vi "UI Main.vi"() -> ()   [LabVIEW 2018]
uses:
  robot state.ctl
  internalstate.ctl
  TrialListElements.ctl
  trial type.ctl
  rewtype.ctl
  frontpanelrobotparams.ctl
  commands.ctl
  DataRecord.ctl
  TrialParams.ctl
  <vilib>/Utility/file.llb/Write Delimited Spreadsheet (DBL).vi
  <resource>/objmgr/ni.dex.rc
panel:
  out "Ready to exit":bool
  in  "nocurrent":bool
  in  "Exit":bool
  in  "Robot\nparameters":T1
  in  "CurrentParams":T2={"TrialType"=enum."2D aiming", "Angle"=0.0, "Length"=0.0, "TurnLength"=0.0, "TurnAngle"=0.0, "MaxError"=0.0, "RewardScale"=0.0, "Timeout"=100, "RewardType"=enum."Normal"} caption="Current trial parameters"
  out "Completed":bool caption="Last trial\ncompleted"
  out "Advance trial":bool
  out "Current reward":u32
  in  "waitforcompletion":bool caption="Wait for \ncompletion"
  out "Last trial rewarded":bool
  in  "AdvanceOnReward":bool=TRUE caption="Only advance\nafter reward"
  in  "Rewarded length":sgl=6.0
  in  "Trial List":T2[](array[typedef]) caption="Upcoming trials"
  in  "Reward":i32=70 caption="Reward (ms)"
  in  "Give reward":bool
  out "Targpos":sgl[](array[numeric])
  in  "Trial list file":path=path "C:/Users/cnc/Desktop/Robot_visual_050319/trial lists/clamp0.csv"
  in  "data file":path=path "C:/Users/cnc/Desktop/junk.csv" caption="Data record file"
  in  "Write data":bool
  out "Last\nmovement":dbl=0.1 caption="Last trial\nradial length" format="%#_2g"
  out "Last lateral\ndeviation":dbl=0.1 caption="Last trial\nlateral length" format="%#.2g"
  out "rewards":i32 caption="# of Rewards"
  in  "Stop block":bool
  out "Xpos":sgl format="%#_3g"
  out "Ypos":sgl=56.0 format="%#_3g"
  in  "Start block":bool
  out "loaded":bool caption="Loaded a\ntrial list"
  out "movement number":i32 caption="Trial #"
  out "Last event":i32 format="%.0e"
  out "UI state":T5
  out "Trial started":bool
  in  "Go to target":bool
  in  "X home":sgl
  in  "Y home":sgl=56.0
  out "Robot state":T6=enum."Go somewhere"
  in  "Hold position":bool
  out "Homing":bool
  in  "Find home":bool
  in  "Go home":bool
  in  "X target":sgl
  in  "Y target":sgl=56.0
  in  "Enable drives":bool
  # "Movement criteria"
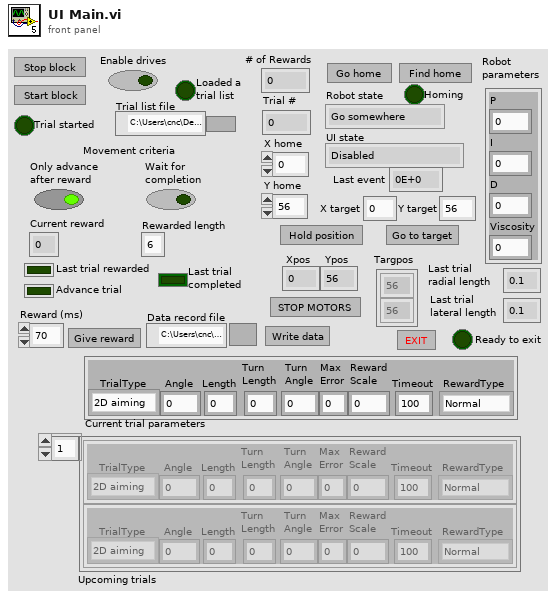
[diagram p1: front panel]
types:
  T1 = typedef "frontpanelrobotparams.ctl" = cluster{"Kp":dbl, "Bp":dbl, "Ip":dbl, "Viscosity":dbl}
  T2 = typedef "TrialListElements.ctl" = cluster{"TrialType":T3, "Angle":dbl, "Length":dbl, "TurnLength":dbl, "TurnAngle":dbl, "MaxError":dbl, "RewardScale":dbl, "Timeout":i32, "RewardType":T4}
  T3 = typedef "trial type.ctl" = enum8{"Linear", "2D aiming", "Two-part"}
  T4 = typedef "rewtype.ctl" = enum16{"Normal", "No reward"}
  T5 = typedef "internalstate.ctl" = enum16{"Disabled", "Waiting for movement", "Moving", "Post-trial", "Returning handle", "Starting trial", "Post-reward"}
  T6 = typedef "robot state.ctl" = enum16{"Hold", "Movement", "Homing", "Go somewhere", "Go home", "Disabled"}
  T7 = typedef "DataRecord.ctl" = cluster{"X":sgl, "Y":sgl, "MotorCurrent1":i16, "MotorCurrent2":i16, "TrialType":T3, "Angle":sgl, "FrameCnt1":i16, "FrameCnt2":i16, "Licking":bool, "Solenoid":bool, "robot state":T6}
  T8 = typedef "commands.ctl" = enum16{"TrialParams", "X home", "Y home", "Target X", "Target Y", "Enable drives", "Robot state", "Shut down", "Reward duration", "Start reward"}
  T9 = typedef "TrialParams.ctl" = cluster{"Kp":dbl, "Bp":dbl, "Ip":dbl, "TrialType":T3, "Angle":dbl, "Viscosity":dbl, "Length":dbl, "MaxError":dbl, "TurnLength":dbl, "TurnAngle":dbl}
  T10 = cluster{"Kp":dbl, "Bp":dbl, "Ip":dbl, "Viscosity":dbl}
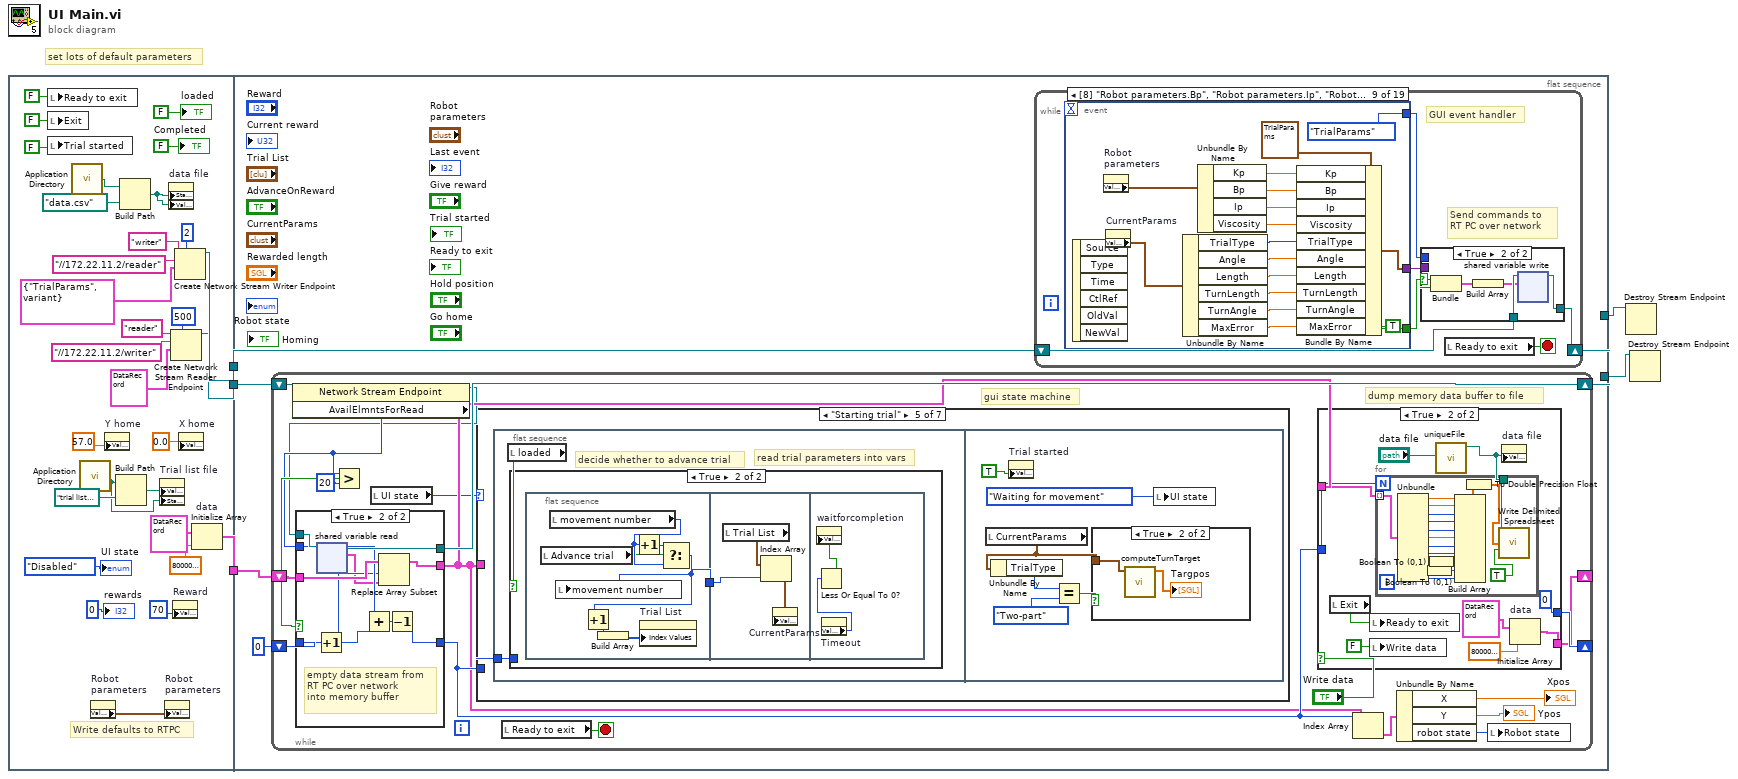
[diagram p0: block diagram]
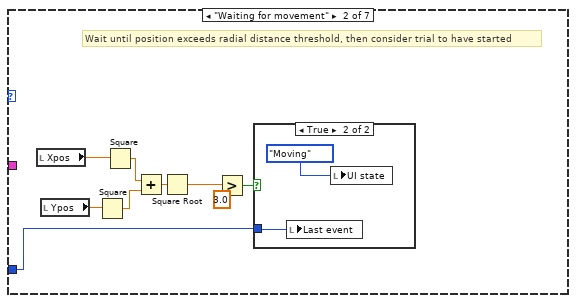
[diagram p3: hidden frame]
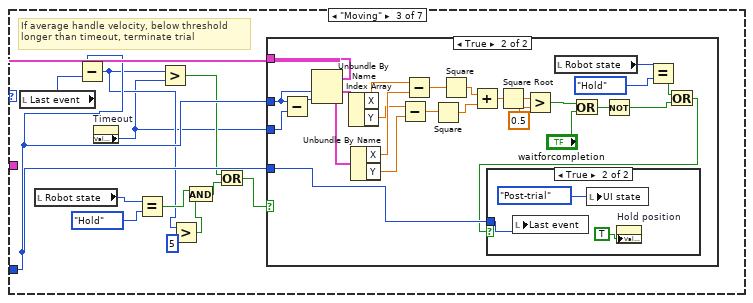
[diagram p5: hidden frame]
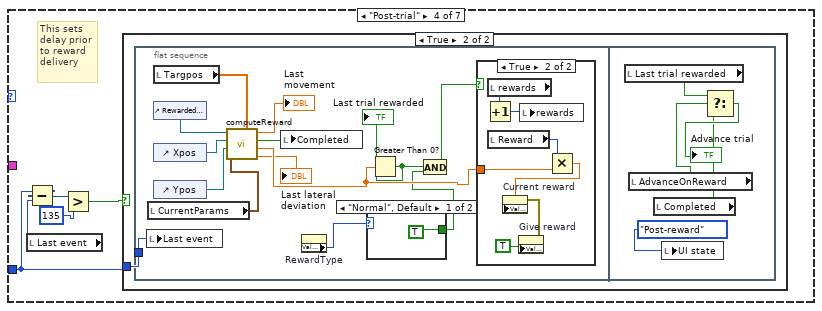
[diagram p8: hidden frame]
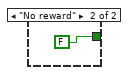
[diagram p10: hidden frame]
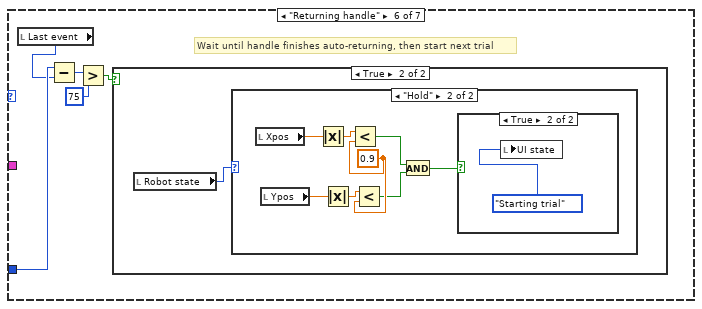
[diagram p14: hidden frame]
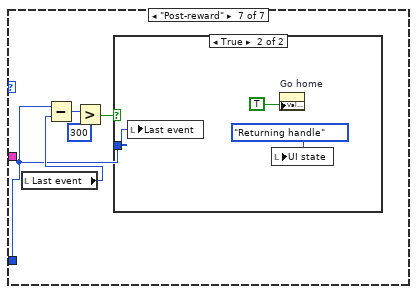
[diagram p18: hidden frame]
diagram:
  # "set lots of default parameters"
  n1 = flat-sequence {
    tunnel: [w28] -> w5
    tunnel: [w27] -> w4
    tunnel: [w25] -> w3
    tunnel: w5 -> [w41]
    tunnel: w4 -> [w40]
    tunnel: [w39] -> w2
    tunnel: w3 -> [w38]
    tunnel: [w36] -> w1
    frame #0 {
      # "Write defaults to RTPC"
      n2 = local write "Ready to exit"(FALSE) -> ()
      n3 = local write "Exit"(FALSE) -> ()
      n4 = local write "Trial started"(FALSE) -> ()
      n5 = call <vilib>:"Application Directory.vi"() -> ("Application Directory"=w19:path)
      n6 = call <vilib>:"Application Directory.vi"() -> ("Application Directory"=w7:path)
      n7 = property on="Robot\nparameters" class="Clust (strict)"() -> ("Value"=w6:T10)  [unwired: 2 in, 2 out]
      n8 = property on="Y home" class="DigNum (strict)"("Val(Sgnl)"=sgl 57.0) -> ()  [unwired: 2 in, 2 out]
      n9 = Build Path(base path=w7, name or relative path=path "trial lists/2D_0deg.csv") -> (appended path=w13:path)
      n10 = Build Path(base path=w19, name or relative path=path "data.csv") -> (appended path=w8:path)
      n11 = property on="Trial list file" class="Path"("Val(Sgnl)"=w13, "StartPath"=w7) -> ()  [unwired: 2 in, 2 out]
      n12 = property on="Robot\nparameters" class="Clust (strict)"("Val(Sgnl)"=w6) -> ()  [unwired: 2 in, 2 out]
      n13 = property on="data file" class="Path"("StartPath"=w8, "Val(Sgnl)"=w8) -> ()  [unwired: 2 in, 2 out]
      n14 = Create Network Stream Reader Endpoint(7:500, 9:T7 {"X"=0.0, "Y"=0.0, "MotorCurrent1"=0, "MotorCurrent2"=0, "TrialType"=enum."Linear", "Angle"=0.0, "FrameCnt1"=0, "FrameCnt2"=0, "Licking"=FALSE, "Solenoid"=FALSE, "robot state"=enum."Go somewhere"} ("DataRecord"), 10:"//172.22.11.2/writer", 11:"reader") -> (3:w27:refnum<k21>)  [unwired: 3 in, 1 out]
      n15 = property on="Reward" class="DigNum (strict)"("Val(Sgnl)"=70) -> ()  [unwired: 2 in, 2 out]
      n16 = Create Network Stream Writer Endpoint(7:2, 9:cluster{"Commands":T8, variant} {"Commands"=enum."TrialParams", variant}, 10:"//172.22.11.2/reader", 11:"writer") -> (3:w28:refnum<k21>)  [unwired: 3 in, 1 out]
      n17 = property on="X home" class="DigNum (strict)"("Val(Sgnl)"=sgl 0.0) -> ()  [unwired: 2 in, 2 out]
      n18 = Initialize Array "data"(T7 {"X"=0.0, "Y"=0.0, "MotorCurrent1"=0, "MotorCurrent2"=0, "TrialType"=enum."Linear", "Angle"=0.0, "FrameCnt1"=0, "FrameCnt2"=0, "Licking"=FALSE, "Solenoid"=FALSE, "robot state"=enum."Go somewhere"} ("DataRecord"), sgl 8000000.0) -> (w25:T7[])
      "loaded" <- FALSE
      "rewards" <- 0
      "Completed" <- FALSE
      "UI state" <- internalstate."Disabled" ("internal state")
    }
    frame #1 {
      n19 = while {
        shift-right: [w59] -> w39
        shift-left: w40 -> [w60]
        shift-right: [w55] -> _
        shift-left: 0 -> [w56]
        shift-right: [w43] -> _
        shift-left: w38 -> [w57]
        stop <- w58 stop-if-true
        # "gui state machine"
        # "dump memory data buffer to file"
        n20 = property class="Network Stream Endpoint"(reference=w60) -> (reference out=w49:refnum<k21>, "AvailElmntsForRead"=w52:i32)  [unwired: 1 in, 1 out]
        n21 = Greater?(x=w52, y=20) -> (0:w53:bool)
        n22 = case shown="True" w53 {
          tunnel: w52 -> [_ w232]
          tunnel: w49 -> [w226 w236]
          tunnel: [w226 w235] -> w59
          tunnel: w57 -> [w225 w234]
          tunnel: w56 -> [w224 w231]
          tunnel: [w225 w233] -> w50
          tunnel: [w224 w228] -> w54
          frame False {
          }
          frame True {
            # "empty data stream from\nRT PC over network\ninto memory buffer"
            n23 = Increment(x=w231) -> (x+1=w229:i32)
            n24 = shared-variable-read(w236, w232) -> (w235:refnum<k21>, w227:T7[])  [unwired: 2 in, 2 out]
            n25 = Add(x=w232, y=w229) -> (x+y=w230:i32)
            n26 = Replace Array Subset(array=w234, new element=w227, index=w229) -> (w233:T7[])
            n27 = Decrement(x=w230) -> (x-1=w228:i32)
          }
        }
        n28 = local read "UI state"() -> (w48:T5)
        n29 = case shown="\"Starting trial\"" w48 {
          tunnel: w50 -> [_ _ w83 _ _ _ _]
          tunnel: w54 -> [_ w64 w82 w115 w148 w174 w186]
          frame "Disabled", Default {
          }
          frame "Waiting for movement" {
            # "Wait until position exceeds radial distance threshold, then consider trial to have started"
            n30 = local read "Xpos"() -> (w62:sgl)
            n31 = local read "Ypos"() -> (w61:sgl)
            n32 = Square(x=w61) -> (x^2=w68:sgl)
            n33 = Square(x=w62) -> (x^2=w69:sgl)
            n34 = Add(x=w69, y=w68) -> (x+y=w67:sgl)
            n35 = Square Root(x=w67) -> (sqrt(x)=w66:sgl)
            n36 = Greater?(x=w66, y=sgl 3.0) -> (0:w63:bool)
            n37 = case shown="True" w63 {
              tunnel: w64 -> [_ w70]
              frame False {
              }
              frame True {
                n38 = local write "Last event"(w70) -> ()
                n39 = local write "UI state"(internalstate."Moving" ("internal state")) -> ()
              }
            }
          }
          frame "Moving" {
            # "If average handle velocity, below threshold \nlonger than timeout, terminate trial"
            n40 = local read "Last event"() -> (w84:i32)
            n41 = local read "Robot state"() -> (w80:T6)
            n42 = Subtract(x=w82, y=w84) -> (x-y=w76:i32)
            n43 = property on="Timeout" class="DigNum (strict)"() -> ("Value"=w72:i32)  [unwired: 2 in, 2 out]
            n44 = Equal?(x=w80, y=robot_state."Hold" ("robot state")) -> (x = y?=w78:bool)
            n45 = Greater?(x=w76, y=w72) -> (0:w79:bool)
            n46 = Greater?(x=w76, y=5) -> (0:w77:bool)
            n47 = And(x=w78, y=w77) -> (x .and. y?=w74:bool)
            n48 = Or(x=w79, y=w74) -> (x .or. y?=w73:bool)
            n49 = case shown="True" w73 {
              tunnel: w83 -> [_ w93]
              tunnel: w72 -> [_ w98]
              tunnel: w82 -> [_ w102]
              tunnel: w82 -> [_ w92]
              frame False {
              }
              frame True {
                n50 = Subtract(x=w92, y=w98) -> (x-y=w91:i32)
                n51 = Index Array(array=w93, index #1=w92, index #2=w91) -> (element #1=w90:T7, element #2=w89:T7)
                n52 = Unbundle By Name(w90) -> ("X"=w87:sgl, "Y"=w86:sgl)
                n53 = Unbundle By Name(w89) -> ("X"=w88:sgl, "Y"=w85:sgl)
                n54 = Subtract(x=w86, y=w85) -> (x-y=w105:sgl)
                n55 = Subtract(x=w87, y=w88) -> (x-y=w104:sgl)
                n56 = Square(x=w105) -> (x^2=w107:sgl)
                n57 = Square(x=w104) -> (x^2=w106:sgl)
                n58 = Add(x=w106, y=w107) -> (x+y=w108:sgl)
                n59 = Square Root(x=w108) -> (sqrt(x)=w109:sgl)
                n60 = Greater?(x=w109, y=sgl 0.5) -> (0:w103:bool)
                n61 = local read "Robot state"() -> (w99:T6)
                n62 = Or(x=w103, y="waitforcompletion") -> (x .or. y?=w95:bool)
                n63 = Not(x=w95) -> (.not. x?=w94:bool)
                n64 = Equal?(x=w99, y=robot_state."Hold" ("robot state")) -> (x = y?=w100:bool)
                n65 = Or(x=w100, y=w94) -> (x .or. y?=w97:bool)
                n66 = case shown="True" w97 {
                  tunnel: w102 -> [_ w112]
                  frame False {
                  }
                  frame True {
                    n67 = local write "Last event"(w112) -> ()
                    n68 = local write "UI state"(internalstate."Post-trial" ("internal state")) -> ()
                    n69 = property on="Hold position" class="Bool (strict)"("Val(Sgnl)"=TRUE) -> ()  [unwired: 2 in, 2 out]
                  }
                }
              }
            }
          }
          frame "Post-trial" {
            # "This sets\ndelay prior\nto reward\ndelivery"
            n70 = local read "Last event"() -> (w118:i32)
            n71 = Subtract(x=w115, y=w118) -> (x-y=w117:i32)
            n72 = Greater?(x=w117, y=135) -> (0:w116:bool)
            n73 = case shown="True" w116 {
              tunnel: w115 -> [_ w119]
              frame False {
              }
              frame True {
                n74 = flat-sequence {
                  tunnel: w119 -> [w130]
                  frame #0 {
                    n75 = local write "Last event"(w130) -> ()
                    n76 = local read "CurrentParams"() -> (w121:T2)
                    n77 = local read "Targpos"() -> (w123:sgl[])
                    n78 = control-ref of="Rewarded length"() -> (w128:refnum<vi>)
                    n79 = control-ref of="Xpos"() -> (w129:refnum<vi>)
                    n80 = control-ref of="Ypos"() -> (w122:refnum<vi>)
                    n81 = call "computeReward.vi"("RewardedLength"=w128, "X"=w129, "Y"=w122, "TrialListElements"=w121, "targpos"=w123) -> ("ylen"=→"Last\nmovement":dbl, "completed"=w126:bool, "reward"=w133:dbl, "xlen"=→"Last lateral\ndeviation":dbl)  [unwired: 2 in]
                    n82 = local write "Completed"(w126) -> ()
                    n83 = property on="RewardType" class="Enum (strict)"() -> ("Value"=w120:T4)  [unwired: 2 in, 2 out]
                    n84 = case shown="\"Normal\", Default" w120 {
                      tunnel: [TRUE FALSE] -> w125
                      frame "Normal", Default {
                      }
                      frame "No reward" {
                      }
                    }
                    n85 = Greater Than 0?(x=w133) -> (x > 0?=w131:bool)
                    "Last trial rewarded" <- w131
                    n86 = And(x=w131, y=w125) -> (x .and. y?=w132:bool)
                    n87 = case shown="True" w132 {
                      tunnel: w133 -> [_ w138]
                      frame False {
                      }
                      frame True {
                        n88 = local read "rewards"() -> (w141:i32)
                        n89 = Increment(x=w141) -> (x+1=w142:i32)
                        n90 = local read "Reward"() -> (w137:i32)
                        n91 = local write "rewards"(w142) -> ()
                        n92 = Multiply(x=w137, y=w138) -> (x*y=w136:dbl)
                        n93 = property on="Current reward" class="DigNum (strict)"("Val(Sgnl)"=w136) -> (error out=w139:errorcluster)  [unwired: 2 in, 1 out]
                        n94 = property on="Give reward" class="Bool (strict)"(error in=w139, "Val(Sgnl)"=TRUE) -> ()  [unwired: 1 in, 2 out]
                      }
                    }
                  }
                  frame #1 {
                    n95 = local read "Last trial rewarded"() -> (w143:bool)
                    n96 = local read "AdvanceOnReward"() -> (w145:bool)
                    n97 = local read "Completed"() -> (w144:bool)
                    n98 = local write "UI state"(internalstate."Post-reward" ("internal state")) -> ()
                    n99 = Select(t=w143, s=w145, f=w144) -> (s? t:f=→"Advance trial":bool)
                  }
                }
              }
            }
          }
          frame "Starting trial" {
            n100 = flat-sequence {
              tunnel: w148 -> [w149]
              frame #0 {
                # "decide whether to advance trial"
                # "read trial parameters into vars"
                n101 = local read "loaded"() -> (w150:bool)
                n102 = case shown="True" w150 {
                  tunnel: w149 -> [_ _]
                  frame False {
                  }
                  frame True {
                    n103 = flat-sequence {
                      tunnel: [w153] -> w151
                      tunnel: w151 -> [w159]
                      frame #0 {
                        n104 = local read "Advance trial"() -> (w152:bool)
                        n105 = local read "movement number"() -> (w156:i32)
                        n106 = Increment(x=w156) -> (x+1=w157:i32)
                        n107 = Select(t=w157, s=w152, f=w156) -> (s? t:f=w153:i32)
                        n108 = local write "movement number"(w153) -> ()
                        n109 = Increment(x=w153) -> (x+1=w154:i32)
                        n110 = Build Array(w154) -> (w155:i32[])
                        n111 = property on="Trial List" class="Arr (strict)"("Index Values"=w155) -> ()  [unwired: 2 in, 2 out]
                      }
                      frame #1 {
                        n112 = local read "Trial List"() -> (w158:T2[])
                        n113 = Index Array(array=w158, index=w159) -> (element=w160:T2)
                        n114 = property on="CurrentParams" class="Clust (strict)"("Val(Sgnl)"=w160) -> ()  [unwired: 2 in, 2 out]
                      }
                      frame #2 {
                        n115 = property on="Timeout" class="DigNum (strict)"() -> ("Value"=w161:i32)  [unwired: 2 in, 2 out]
                        n116 = Less Or Equal To 0?(x=w161) -> (x <= 0?=w162:bool)
                        n117 = property on="waitforcompletion" class="Bool (strict)"("Val(Sgnl)"=w162) -> ()  [unwired: 2 in, 2 out]
                      }
                    }
                  }
                }
              }
              frame #1 {
                n118 = local read "CurrentParams"() -> (w163:T2)
                n119 = Unbundle By Name(w163) -> ("TrialType"=w164:T3)
                n120 = property on="Trial started" class="Bool (strict)"("Val(Sgnl)"=TRUE) -> ()  [unwired: 2 in, 2 out]
                n121 = Equal?(x=w164, y=trial_type."Two-part" ("Enum")) -> (x = y?=w167:bool)
                n122 = case shown="True" w167 {
                  tunnel: w163 -> [_ w169]
                  frame False {
                  }
                  frame True {
                    n123 = call "computeTurnTarget.vi"("Cluster in"=w169) -> ("Targpos"=→"Targpos":sgl[])  [unwired: 10 in]
                  }
                }
                n124 = local write "UI state"(internalstate."Waiting for movement" ("internal state")) -> ()
              }
            }
          }
          frame "Returning handle" {
            # "Wait until handle finishes auto-returning, then start next trial"
            n125 = local read "Last event"() -> (w173:i32)
            n126 = Subtract(x=w174, y=w173) -> (x-y=w172:i32)
            n127 = Greater?(x=w172, y=75) -> (0:w171:bool)
            n128 = case shown="True" w171 {
              frame False {
              }
              frame True {
                n129 = local read "Robot state"() -> (w176:T6)
                n130 = case shown="\"Hold\"" w176 {
                  frame "Go home", Default {
                  }
                  frame "Hold" {
                    w180 = 0.9
                    n131 = local read "Xpos"() -> (w184:sgl)
                    n132 = local read "Ypos"() -> (w183:sgl)
                    n133 = Absolute Value(x=w184) -> (abs(x)=w182:sgl)
                    n134 = Absolute Value(x=w183) -> (abs(x)=w181:sgl)
                    n135 = Less?(x=w182, y=w180) -> (x < y?=w179:bool)
                    n136 = Less?(x=w181, y=w180) -> (x < y?=w178:bool)
                    n137 = And(x=w179, y=w178) -> (x .and. y?=w177:bool)
                    n138 = case shown="True" w177 {
                      frame False {
                      }
                      frame True {
                        n139 = local write "UI state"(internalstate."Starting trial" ("internal state")) -> ()
                      }
                    }
                  }
                }
              }
            }
          }
          frame "Post-reward" {
            n140 = local read "Last event"() -> (w189:i32)
            n141 = Subtract(x=w186, y=w189) -> (x-y=w188:i32)
            n142 = Greater?(x=w188, y=300) -> (0:w187:bool)
            n143 = case shown="True" w187 {
              tunnel: w186 -> [_ w193]
              frame False {
              }
              frame True {
                n144 = local write "Last event"(w193) -> ()
                n145 = local write "UI state"(internalstate."Returning handle" ("internal state")) -> ()
                n146 = property on="Go home" class="Bool (strict)"("Val(Sgnl)"=TRUE) -> ()  [unwired: 2 in, 2 out]
              }
            }
          }
        }
        n147 = local read "Ready to exit"() -> (w58:bool)
        n148 = case shown="True" "Write data" {
          tunnel: w50 -> [w194 w199]
          tunnel: [w194 w201] -> w43
          tunnel: [w195 0] -> w55
          tunnel: w54 -> [w195 w197]
          frame False {
          }
          frame True {
            n149 = local read "Exit"() -> (w198:bool)
            n150 = local write "Ready to exit"(w198) -> ()
            n151 = local write "Write data"(FALSE) -> ()
            n152 = call "uniqueFile.vi"("PathIn"="data file") -> ("PathOut"=w196:path)  [unwired: 10 in]
            n153 = for {
              N: w197 -> [_]
              tunnel: w199 -> [w223] mode=indexing
              tunnel: w196 -> [w208]
              n154 = Unbundle(w223) -> ("X"=w222:sgl, "Y"=w221:sgl, "MotorCurrent1"=w220:i16, "MotorCurrent2"=w219:i16, "TrialType"=w218:T3, "Angle"=w217:sgl, "FrameCnt1"=w216:i16, "FrameCnt2"=w215:i16, "Licking"=w214:bool, "Solenoid"=w212:bool, "robot state"=w210:T6)
              n155 = Boolean To (0,1)(Boolean=w212) -> (0, 1=w211:i16)
              n156 = Boolean To (0,1)(Boolean=w214) -> (0, 1=w213:i16)
              n157 = Build Array(w222, w221, w220, w219, w218, w217, w216, w215, w213, w211, w210) -> (w209:sgl[])
              n158 = To Double Precision Float(number=w209) -> (double precision float=w207:dbl[])
              n159 = call-poly <vilib>:"Write Delimited Spreadsheet.vi"("file path (dialog if empty)"=w208, "1D data"=w207, "append to file? (new file:F)"=TRUE) -> ()  [unwired: 11 in, 2 out]
            }
            n160 = property on="data file" class="Path"("Val(Sgnl)"=w196) -> ()  [unwired: 2 in, 2 out]
            n161 = Initialize Array "data"(T7 {"X"=0.0, "Y"=0.0, "MotorCurrent1"=0, "MotorCurrent2"=0, "TrialType"=enum."Linear", "Angle"=0.0, "FrameCnt1"=0, "FrameCnt2"=0, "Licking"=FALSE, "Solenoid"=FALSE, "robot state"=enum."Go somewhere"} ("DataRecord"), sgl 8000000.0) -> (w201:T7[])
          }
        }
        n162 = Index Array(array=w50, index=w54) -> (element=w47:T7)
        n163 = Unbundle By Name(w47) -> ("X"=→"Xpos":sgl, "Y"=→"Ypos":sgl, "robot state"=w46:T6)
        n164 = local write "Robot state"(w46) -> ()
      }
      n165 = while {
        shift-right: [w239] -> w36
        shift-left: w41 -> [w242]
        stop <- w238 stop-if-true
        # "GUI event handler"
        # "Send commands to \nRT PC over network"
        n166 = event shown="[8] \"Robot parameters.Bp\", \"Robot parameters.Ip\", \"Robot parameters.Viscosity\", \"CurrentParams.Length\", \"CurrentParams.RewardScale\", \"CurrentParams.TrialType\", \"CurrentParams.Angle\", \"CurrentParams.TurnLength\", \"CurrentParams.TurnAngle\", \"CurrentParams.MaxError\": Value Change" {
          selector: _ -> [_ _ _ _ _ _ _ _ _ _ _ _ _ _ _ _ _ _ _]
          dyn-events: _ -> [_ _ _ _ _ _ _ _ _ _ _ _ _ _ _ _ _ _ _]
          timeout: _ -> [_ _ _ _ _ _ _ _ _ _ _ _ _ _ _ _ _ _ _]
          tunnel: ["Enable drives" robot_state."Go somewhere" ("robot state") robot_state."Movement" ("robot state") "X home" "Y home" TRUE w272 _ w276 w293 _ "X target" "Y target" robot_state."Go home" ("robot state") robot_state."Homing" ("robot state") robot_state."Hold" ("robot state") _ _ _] -> w240
          tunnel: [commands."Enable drives" ("Commands") commands."Robot state" ("Commands") commands."Robot state" ("Commands") commands."X home" ("Commands") commands."Y home" ("Commands") commands."Start reward" ("Commands") commands."Reward duration" ("Commands") _ commands."TrialParams" ("Commands") commands."Robot state" ("Commands") _ commands."Target X" ("Commands") commands."Target Y" ("Commands") commands."Robot state" ("Commands") commands."Robot state" ("Commands") commands."Robot state" ("Commands") _ _ _] -> w241
          tunnel: [TRUE TRUE TRUE TRUE TRUE TRUE TRUE FALSE TRUE TRUE _ TRUE TRUE TRUE TRUE TRUE FALSE FALSE FALSE] -> w237
          event "Enable drives": Value Change {
            n167 = event-data() -> ()  [unwired: 1 in, 5 out]
          }
          event "Go to target": Value Change {
            n168 = event-data() -> ()  [unwired: 1 in, 1 out]
          }
          event "Trial started": Value Change {
            n169 = event-data() -> ()  [unwired: 1 in, 5 out]
            n170 = local write "Trial started"(FALSE) -> ()
          }
          event "X home": Value Change {
            n171 = event-data() -> ()  [unwired: 1 in, 5 out]
          }
          event "Y home": Value Change {
            n172 = event-data() -> ()  [unwired: 1 in, 5 out]
          }
          event "Give reward": Value Change {
            n173 = event-data() -> ()  [unwired: 1 in, 6 out]
            n174 = local write "Give reward"(FALSE) -> ()
          }
          event "Current reward": Value Change {
            n175 = event-data() -> ()  [unwired: 1 in, 6 out]
            n176 = local read "Current reward"() -> (w272:u32)
          }
          event "Reward": Value Change {
            n177 = event-data() -> ()  [unwired: 1 in, 6 out]
            n178 = local read "Reward"() -> (w273:i32)
            n179 = control-ref of="Current reward"() -> (w274:refnum<vi>)
            n180 = property class="DigNum (strict)"(reference=w274, "Val(Sgnl)"=w273) -> ()  [unwired: 1 in, 2 out]
          }
          event Value Change {
            n181 = event-data() -> ()  [unwired: 1 in, 6 out]
            n182 = property on="Robot\nparameters" class="Clust (strict)"() -> ("Value"=w288:T10)  [unwired: 2 in, 2 out]
            n183 = property on="CurrentParams" class="Clust (strict)"() -> ("Value"=w283:T2)  [unwired: 2 in, 2 out]
            n184 = Unbundle By Name(w283) -> ("TrialType"=w282:T3, "Angle"=w281:dbl, "Length"=w280:dbl, "TurnLength"=w279:dbl, "TurnAngle"=w278:dbl, "MaxError"=w277:dbl)
            n185 = Unbundle By Name(w288) -> ("Kp"=w287:dbl, "Bp"=w286:dbl, "Ip"=w285:dbl, "Viscosity"=w284:dbl)
            n186 = Bundle By Name(cluster=T9 {"Kp"=0.0, "Bp"=0.0, "Ip"=0.0, "TrialType"=enum."Linear", "Angle"=0.0, "Viscosity"=0.0, "Length"=0.0, "MaxError"=0.0, "TurnLength"=0.0, "TurnAngle"=0.0} ("TrialParams"), "Kp"=w287, "Bp"=w286, "Ip"=w285, "Viscosity"=w284, "TrialType"=w282, "Angle"=w281, "Length"=w280, "TurnLength"=w279, "TurnAngle"=w278, "MaxError"=w277) -> (w276:T9)
          }
          event "nocurrent": Value Change {
            n187 = event-data() -> ()  [unwired: 1 in, 6 out]
            n188 = local write "UI state"(internalstate."Disabled" ("internal state")) -> ()
            n189 = To Variant(anything=robot_state."Disabled" ("robot state")) -> (Variant=w293:variant)
          }
          event "Exit": Value Change {
            n190 = event-data() -> ()  [unwired: 1 in, 6 out]
            n191 = property on="Write data" class="Bool (strict)"("Val(Sgnl)"="Exit") -> ()  [unwired: 2 in, 2 out]
          }
          event "X target": Value Change {
            n192 = event-data() -> ()  [unwired: 1 in, 5 out]
          }
          event "Y target": Value Change {
            n193 = event-data() -> ()  [unwired: 1 in, 5 out]
          }
          event "Go home": Value Change {
            n194 = event-data() -> ()  [unwired: 1 in, 5 out]
            n195 = local write "Go home"(FALSE) -> ()
          }
          event "Find home": Value Change {
            n196 = event-data() -> ()  [unwired: 1 in, 5 out]
          }
          event "Hold position": Value Change {
            n197 = event-data() -> ()  [unwired: 1 in, 5 out]
            n198 = local write "Hold position"(FALSE) -> ()
          }
          event "Trial list file": Value Change {
            n199 = event-data() -> ()  [unwired: 1 in, 1 out]
            n200 = call "ReadTrialList.vi"("InputList"="Trial list file") -> ("TrialList"=w315:T2[])  [unwired: 10 in]
            n201 = local write "loaded"(TRUE) -> ()
            n202 = property on="Trial List" class="Arr (strict)"("Value"=w315) -> ()  [unwired: 2 in, 2 out]
            "movement number" <- 0
          }
          event "Stop block": Value Change {
            n203 = event-data() -> ()  [unwired: 1 in, 1 out]
            n204 = property on="Hold position" class="Bool (strict)"("Val(Sgnl)"=TRUE) -> ()  [unwired: 2 in, 2 out]
            n205 = local write "UI state"(internalstate."Disabled" ("internal state")) -> ()
          }
          event "Start block": Value Change {
            n206 = event-data() -> ()  [unwired: 1 in, 1 out]
            n207 = local write "UI state"(internalstate."Starting trial" ("internal state")) -> ()
          }
        }
        n208 = case shown="True" w237 {
          tunnel: w242 -> [w243 w249]
          tunnel: w241 -> [_ w248]
          tunnel: w240 -> [_ w247]
          tunnel: [w243 w245] -> w239
          frame False {
          }
          frame True {
            n209 = Bundle("Commands"=w248, "Variant"=w247) -> (w246:cluster{"Commands":T8, "Variant":variant})  [unwired: 1 in]
            n210 = Build Array(w246) -> (w244:cluster{"Commands":T8, "Variant":variant}[])
            n211 = shared-variable-write(w249, w244) -> (w245:refnum<k21>)  [unwired: 2 in, 2 out]
          }
        }
        n212 = local read "Ready to exit"() -> (w238:bool)
      }
    }
  }
  n213 = Destroy Stream Endpoint(11:w1) -> ()  [unwired: 1 in, 1 out]
  n214 = Destroy Stream Endpoint(11:w2) -> ()  [unwired: 1 in, 1 out]
